vi "Handle Server Request.vi"(8 "error in (no error)":errorcluster, 10 "Request":T1, 11 "Server in":refnum<class "Server.lvclass">) -> (0 "error out":errorcluster, 1 "Protocol Error":errorcluster, 2 "ServerResponse":refnum<class "ControlPacket.lvclass">, 3 "Server out":refnum<class "Server.lvclass">)   [LabVIEW 2013, in "MQTT Server.lvlib" / "Server.lvclass"]
uses:
  Server.lvclass
  Request -- cluster.ctl
  Control Packets/ControlPacket/ControlPacket.lvclass
  Response -- cluster.ctl
  Control Packets/CONNECT/CONNECT.lvclass
  Control Packets/CONNACK/Connect Return Code -- enum.ctl
  Control Packets/CONNACK/CONNACK.lvclass
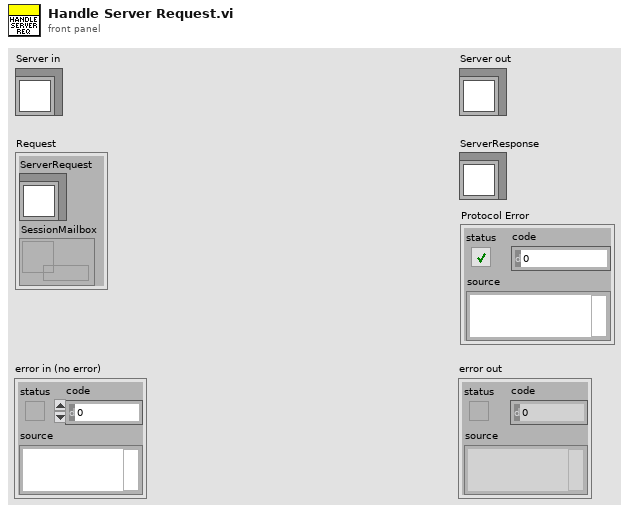
[diagram p1: front panel]
types:
  T1 = typedef "MQTT Server.lvlib/Server.lvclass/Request -- cluster.ctl" = cluster{"ServerRequest":refnum<class "ControlPacket.lvclass">, "SessionMailbox":refnum<queue>}
  T2 = typedef "CONNACK.lvclass/Connect Return Code -- enum.ctl" = enum16{"Connection accepted", "Unacceptable protocol version", "Identifier Rejected", "Server Unavailable", "Bad Username or Password", "Not Authorized"}
  T3 = typedef "ControlPacket.lvclass/Control Packet Type -- enum.ctl" = enum16{"Reserved", "CONNECT", "CONNACK", "PUBLISH", "PUBACK", "PUBREC", "PUBREL", "PUBCOMP", "SUBSCRIBE", "SUBACK", "UNSUBSCRIBE", "UNSUBACK", "PINGREQ", "PINGRESP", "DISCONNECT", "Reserved(15)"}
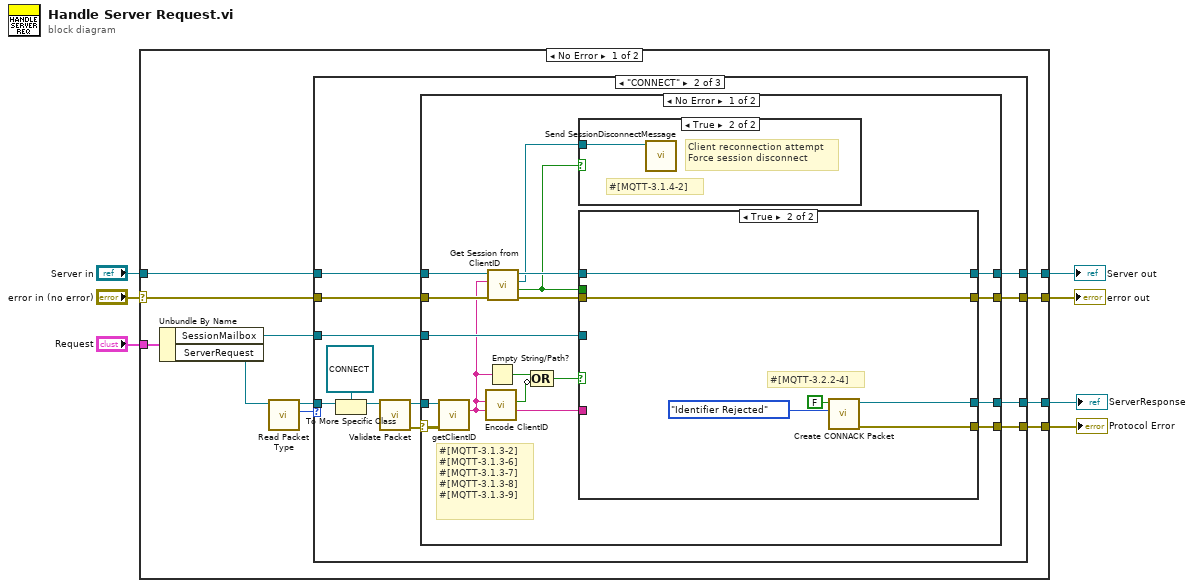
[diagram p0: block diagram]
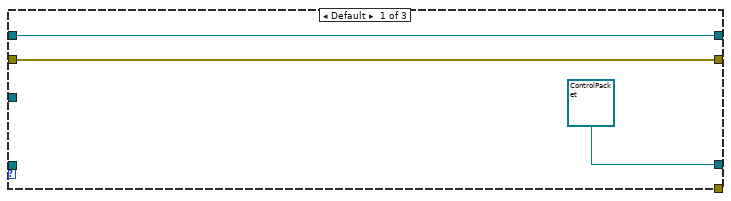
[diagram p2: hidden frame]
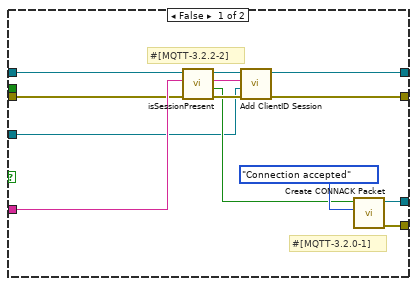
[diagram p4: hidden frame]
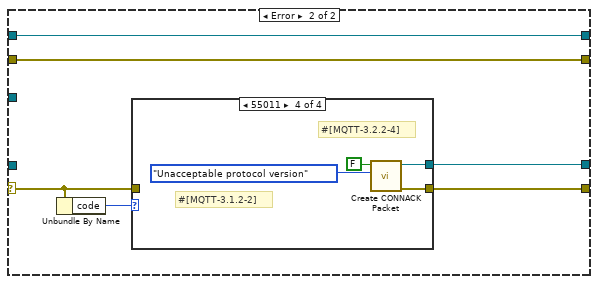
[diagram p5: hidden frame]
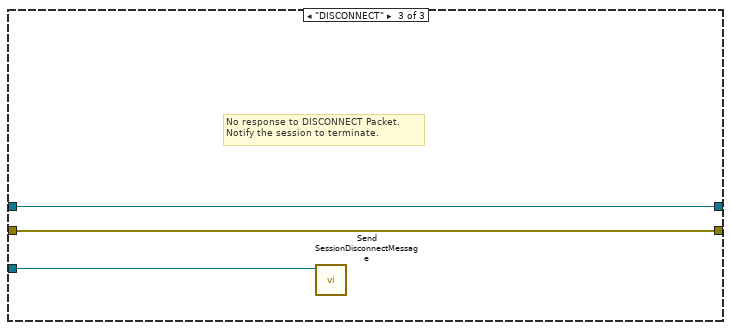
[diagram p9: hidden frame]
diagram:
  n1 = case shown="No Error" "error in (no error)" {
    selector: "error in (no error)" -> [w16 w87]
    tunnel: [w13 w87] -> w6
    tunnel: [w14 w86] -> w4
    tunnel: "Server in" -> [w15 w86]
    tunnel: "Request" -> [w12 _]
    tunnel: [w9 _] -> w2
    tunnel: [w8 _] -> w1
    frame No Error {
      n2 = Unbundle By Name(w12) -> ("SessionMailbox"=w10:refnum<queue>, "ServerRequest"=w11:refnum<class "ControlPacket.lvclass">)
      n3 = call "Read Packet Type.vi"("ControlPacket in"=w11) -> ("Control Packet Type"=w18:T3, "ControlPacket out"=w17:refnum<class "ControlPacket.lvclass">)  [unwired: 9 in]
      n4 = case shown="\"CONNECT\"" w18 {
        tunnel: w17 -> [_ w30 _]
        tunnel: w16 -> [w20 w27 w84]
        tunnel: w15 -> [w21 w28 w85]
        tunnel: [w21 w25 w85] -> w14
        tunnel: [w20 w26 w84] -> w13
        tunnel: w10 -> [_ w24 w83]
        tunnel: [refnum<class "ControlPacket.lvclass"> refnum ("ServerResponse") w23 _] -> w9
        tunnel: [_ w22 _] -> w8
        frame Default {
        }
        frame "CONNECT" {
          n5 = To More Specific Class(target class=refnum<class "CONNECT.lvclass"> refnum ("CONNECT.lvclass"), reference=w30) -> (specific class reference=w29:refnum<class "CONNECT.lvclass">)  [unwired: 1 in, 1 out]
          n6 = call "Validate Packet.vi"("ControlPacket in"=w29) -> ("error out"=w33:errorcluster, "ControlPacket out"=w32:refnum<class "CONNECT.lvclass">)  [unwired: 9 in]
          n7 = case shown="No Error" w33 {
            selector: w33 -> [_ w74]
            tunnel: w32 -> [w49 _]
            tunnel: w28 -> [w45 w73]
            tunnel: w27 -> [w43 w72]
            tunnel: [w47 w72] -> w26
            tunnel: [w48 w73] -> w25
            tunnel: w24 -> [w46 _]
            tunnel: [w36 w71] -> w23
            tunnel: [w35 w70] -> w22
            frame No Error {
              # "#[MQTT-3.1.3-2]\n#[MQTT-3.1.3-6]\n#[MQTT-3.1.3-7]\n#[MQTT-3.1.3-8]\n#[MQTT-3.1.3-9]"
              n8 = call "getClientID.vi"("CONNECT in"=w49) -> ("Client ID"=w39:string)  [unwired: 9 in, 1 out]
              n9 = call "Encode ClientID.vi"("Client ID (empty: generate new)"=w39) -> ("valid Client ID"=w38:bool)  [unwired: 9 in, 1 out]
              n10 = Empty String/Path?(string/path=w39) -> (empty?=w41:bool)
              n11 = call "Get Session from ClientID.vi"("error in (no error)"=w43, "Client ID"=w39, "Server in"=w45) -> ("error out"=w42:errorcluster, "found?"=w34:bool, "SessionMailbox"=w37:refnum<queue>, "Server out"=w44:refnum<class "Server.lvclass">)  [unwired: 5 in]
              n12 = Compound Arithmetic op=OR(w41, invert w38) -> (w40:bool)
              n13 = case shown="True" w34 {
                tunnel: w37 -> [_ w50]
                frame False {
                }
                frame True {
                  # "#[MQTT-3.1.4-2]"
                  # "Client reconnection attempt\nForce session disconnect"
                  n14 = call "Send SessionDisconnectMessage.vi"("SessionMailbox"=w50) -> ()  [unwired: 10 in, 1 out]
                }
              }
              n15 = case shown="True" w40 {
                tunnel: [w62 w67] -> w48
                tunnel: [w61 w66] -> w47
                tunnel: w46 -> [w51 _]
                tunnel: w44 -> [w53 w67]
                tunnel: w42 -> [w52 w66]
                tunnel: w39 -> [w57 _]
                tunnel: [w60 w65] -> w36
                tunnel: [w59 w64] -> w35
                tunnel: w34 -> [_ _]
                frame False {
                  # "#[MQTT-3.2.2-2]"
                  # "#[MQTT-3.2.0-1]"
                  n16 = call "isSessionPresent.vi"("error in"=w52, "Client ID"=w57, "Server in"=w53) -> ("error out"=w58:errorcluster, "Session Present"=w55:bool, "Client ID dup"=w56:string, "Server out"=w54:refnum<class "Server.lvclass">)  [unwired: 5 in]
                  n17 = call "Add ClientID Session.vi"("error in (no error)"=w58, "SessionMailbox"=w51, "Client ID"=w56, "Server in"=w54) -> ("error out"=w61:errorcluster, "Server out"=w62:refnum<class "Server.lvclass">)  [unwired: 6 in]
                  n18 = call "Create CONNACK Packet.vi"("Return Code"=Connect_Return_Code_--_enum."Connection accepted", "Session Present"=w55) -> ("error out"=w59:errorcluster, "CONNACK"=w60:refnum<class "CONNACK.lvclass">)  [unwired: 8 in]
                }
                frame True {
                  # "#[MQTT-3.2.2-4]"
                  n19 = call "Create CONNACK Packet.vi"("Return Code"=Connect_Return_Code_--_enum."Identifier Rejected", "Session Present"=FALSE) -> ("error out"=w64:errorcluster, "CONNACK"=w65:refnum<class "CONNACK.lvclass">)  [unwired: 8 in]
                }
              }
            }
            frame Error {
              n20 = Unbundle By Name(w74) -> ("code"=w75:i32)
              n21 = case shown="55011" w75 {
                tunnel: [_ _ _ w80] -> w71
                tunnel: [w76 w77 w78 w79] -> w70
                tunnel: w74 -> [w76 w77 w78 _]
                frame Default {
                  # "#[MQTT-3.1.4-1]"
                  # "Any unhandled error should be\nthralled to the Protocol error terminal"
                }
                frame 55010 {
                  # "#[MQTT-3.1.2-1]"
                }
                frame 55012 {
                  # "#[MQTT-3.1.2-3]"
                }
                frame 55011 {
                  # "#[MQTT-3.2.2-4]"
                  # "#[MQTT-3.1.2-2]"
                  n22 = call "Create CONNACK Packet.vi"("Return Code"=Connect_Return_Code_--_enum."Unacceptable protocol version", "Session Present"=FALSE) -> ("error out"=w79:errorcluster, "CONNACK"=w80:refnum<class "CONNACK.lvclass">)  [unwired: 8 in]
                }
              }
            }
          }
        }
        frame "DISCONNECT" {
          # "No response to DISCONNECT Packet.\nNotify the session to terminate."
          n23 = call "Send SessionDisconnectMessage.vi"("SessionMailbox"=w83) -> ()  [unwired: 10 in, 1 out]
        }
      }
    }
    frame Error {
    }
  }
  "error out" <- w6
  "Server out" <- w4
  "ServerResponse" <- w2
  "Protocol Error" <- w1
